vi "NI VeriStand - Get Custom Device Channel Data.vi"(8 "error in (no error)":errorcluster, 11 "Channel Ref in":T3 format="%.0x") -> (0 "error out":errorcluster, 1 "Channel":T1, 2 "Channel Name":string, 3 "Channel Ref out":T3 format="%.0x", 4 "Found":bool, 5 "GUID":string)   [LabVIEW 2026, in "Custom Devices Storage.lvlib"]
uses:
  Custom Devices Storage.lvlib
  <vilib>/NI VeriStand/Custom Device API/Custom Device Item Ref.ctl
  <vilib>/NI VeriStand/Custom Device API/Custom Device Channel.ctl
  <vilib>/NI VeriStand/Custom Device API/Custom Device Channel Type.ctl
  C:/Users/Administrator/Desktop/Jatin/All DNC DLLs/NationalInstruments.VeriStand.SystemDefinitionAPI.dll
  Jatin/All DNC DLLs/NationalInstruments.VeriStand.SystemDefinitionAPI.dll
  <vilib>/NI VeriStand/Custom Device API/Custom Device API.lvlib
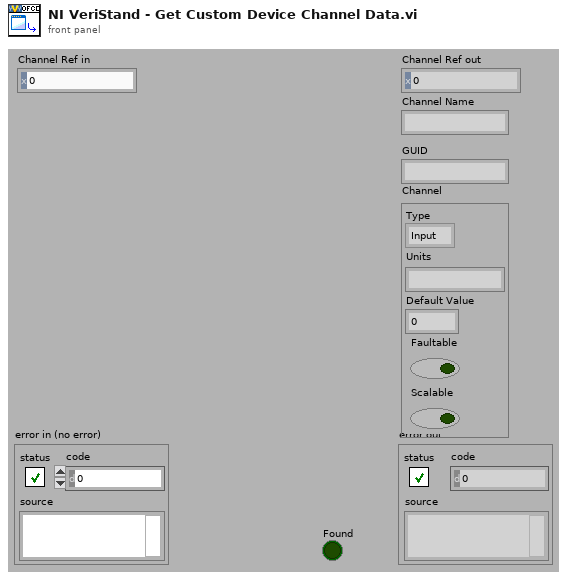
[diagram p1: front panel]
types:
  T1 = typedef "Custom Device API.lvlib/Custom Device Channel.ctl" = cluster{"Type":T2, "Units":string, "Default Value":dbl, "Faultable":bool, "Scalable":bool}
  T2 = typedef "Custom Device API.lvlib/Custom Device Channel Type.ctl" = enum16{"Input", "Output"}
  T3 = typedef "Custom Device API.lvlib/Custom Device Item Ref.ctl" = u64
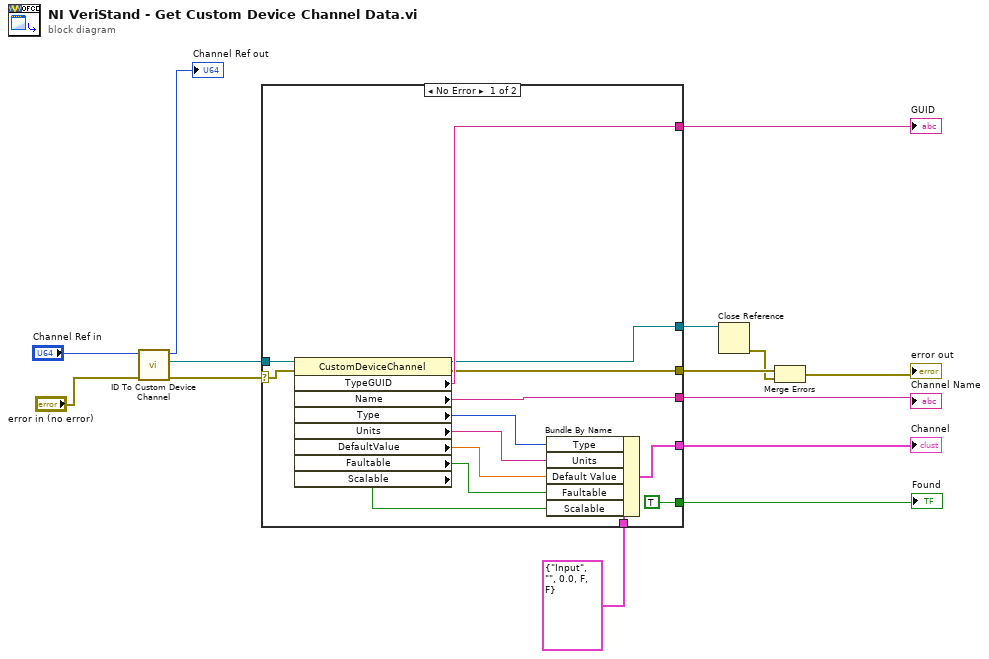
[diagram p0: block diagram]
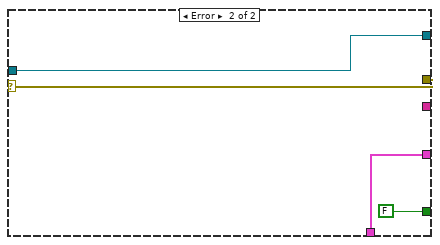
[diagram p2: hidden frame]
diagram:
  n1 = call "ID To Custom Device Channel.vi"("error in (no error)"="error in (no error)", "ID in"="Channel Ref in") -> ("error out"=w12:errorcluster, "NationalInstruments.VeriStand.SystemDefinitionAPI.CustomDeviceChannel"=w11:refnum<k39>, "ID out"=→"Channel Ref out":u64)  [unwired: 7 in]
  n2 = case shown="No Error" w12 {
    selector: w12 -> [w26 w30]
    tunnel: w11 -> [w28 w29]
    tunnel: [w27 _] -> w9
    tunnel: [w25 w30] -> w8
    tunnel: [w24 _] -> w7
    tunnel: [TRUE FALSE] -> w6
    tunnel: [w21 w31] -> w5
    tunnel: T1 {"Type"=enum."Input", "Units"="", "Default Value"=0.0, "Faultable"=FALSE, "Scalable"=FALSE} ("Channel") -> [w22 w31]
    tunnel: [w15 w29] -> w3
    frame No Error {
      n3 = property class="CustomDeviceChannel"(reference=w28, error in=w26) -> (reference out=w15:refnum<k39>, error out=w25:errorcluster, "TypeGUID"=w27:string, "Name"=w24:string, "Type"=w20:i32, "Units"=w19:string, "DefaultValue"=w18:dbl, "Faultable"=w17:bool, "Scalable"=w16:bool)
      n4 = Bundle By Name(cluster=w22, "Type"=w20, "Units"=w19, "Default Value"=w18, "Faultable"=w17, "Scalable"=w16) -> (w21:T1)
    }
    frame Error {
    }
  }
  "Channel" <- w5
  "Found" <- w6
  "GUID" <- w9
  "Channel Name" <- w7
  n5 = Close Reference(reference=w3) -> (error out=w1:errorcluster)  [unwired: 1 in]
  n6 = Merge Errors(w8, w1) -> (→"error out":errorcluster)
